vi "FilterWheelMove.vi"(8 "error in (no error)":errorcluster, 10 "Filter Configuraton":u16, 11 "hdl in":i32) -> (0 "error out":errorcluster, 1 "Get Position":i32, 3 "hdl out":i32)   [LabVIEW 2023]
uses:
  <instrlib>/Thorlabs_FWxC/Thorlabs_FWxC.lvlib
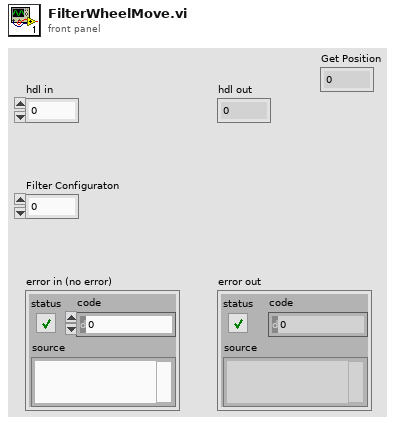
[diagram p1: front panel]
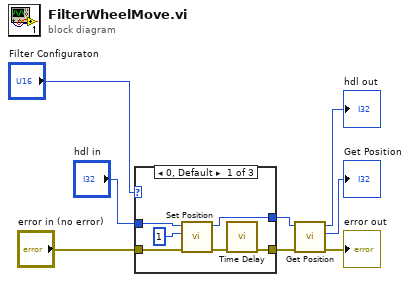
[diagram p0: block diagram]
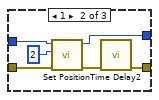
[diagram p2: hidden frame]
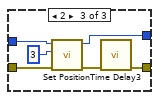
[diagram p3: hidden frame]
diagram:
  n1 = case shown="0, Default" "Filter Configuraton" {
    tunnel: "hdl in" -> [w14 w19 w25]
    tunnel: "error in (no error)" -> [w9 w15 w23]
    tunnel: [w11 w17 w21] -> w5
    tunnel: [w10 w16 w24] -> w2
    frame 0, Default {
      n2 = call <instrlib>:"Set Position.vi"("error in (no error)"=w9, "Set Position"=1, "hdl in"=w14) -> ("error out"=w12:errorcluster, "hdl out"=w10:i32)  [unwired: 7 in]
      n3 = call "Time Delay"("error in (no error)"=w12) -> ("error out"=w11:errorcluster)  [unwired: 10 in]
    }
    frame 1 {
      n4 = call <instrlib>:"Set Position.vi"("error in (no error)"=w15, "Set Position"=2, "hdl in"=w19) -> ("error out"=w18:errorcluster, "hdl out"=w16:i32)  [unwired: 7 in]
      n5 = call "Time Delay2"("error in (no error)"=w18) -> ("error out"=w17:errorcluster)  [unwired: 10 in]
    }
    frame 2 {
      n6 = call <instrlib>:"Set Position.vi"("error in (no error)"=w23, "Set Position"=3, "hdl in"=w25) -> ("error out"=w22:errorcluster, "hdl out"=w24:i32)  [unwired: 7 in]
      n7 = call "Time Delay3"("error in (no error)"=w22) -> ("error out"=w21:errorcluster)  [unwired: 10 in]
    }
  }
  n8 = call <instrlib>:"Get Position.vi"("error in (no error)"=w5, "hdl in"=w2) -> ("error out"=→"error out":errorcluster, "Get Position"=→"Get Position":i32, "hdl out"=→"hdl out":i32)  [unwired: 7 in]
